vi "Init.vi"(8 "error in":errorcluster, 11 "Acquire Continuous Waveform Configuration in":refnum<class "Continuous Waveform Acq CFG.lvclass">) -> (0 "error out":errorcluster, 3 "Acquire Continuous Waveform Configuration out":refnum<class "Continuous Waveform Acq CFG.lvclass">)   [LabVIEW 2023, in "RIGOL DS1054.lvlib" / "Continuous Waveform Acq CFG.lvclass"]
uses:
  Continuous Waveform Acq CFG.lvclass
  <instrlib>/RIGOL DS1000 Series/RIGOL DS1000 Series.lvlib
  Configuration Base/Configuration Base.lvclass
  a845dea6-c2f2-4e03-ac8d-35208e94dd6c.vi
  <vilib>/ErrorRing/Error Ring.xnode
  <vilib>/Utility/error.llb/Error Cluster From Error Code.vi
  Scope VISA/Configuration/Scope VISA CFG.lvclass
  D:/git/HAL/Scope VISA/Configuration/Scope VISA CFG.lvclass
  D:/git/HAL/Scope Base/Configuration/Scope Base CFG.lvclass
  D:/git/HAL/Configuration Base/Configuration Base.lvclass
  D:/git/HAL/Interfaces/IConfigure/IConfigure.lvclass
  D:/git/HAL/Devices/Rigol DS1054/Configurations/Acquire Continuous Waveform/Continuous Waveform Acq CFG.lvclass
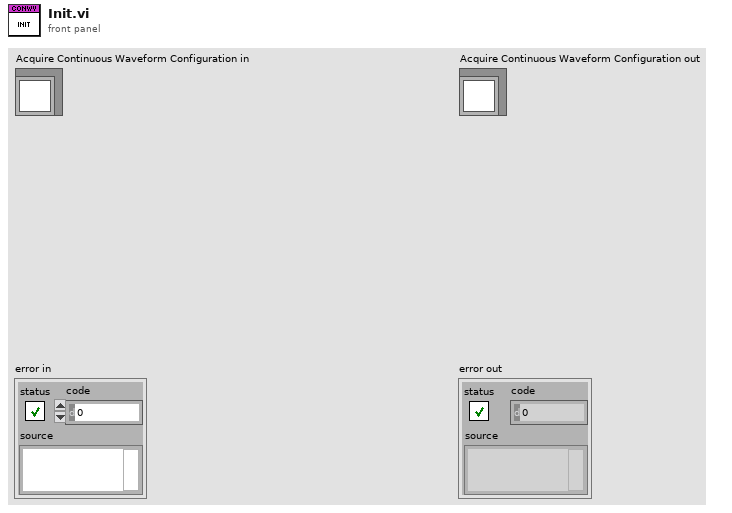
[diagram p1: front panel]
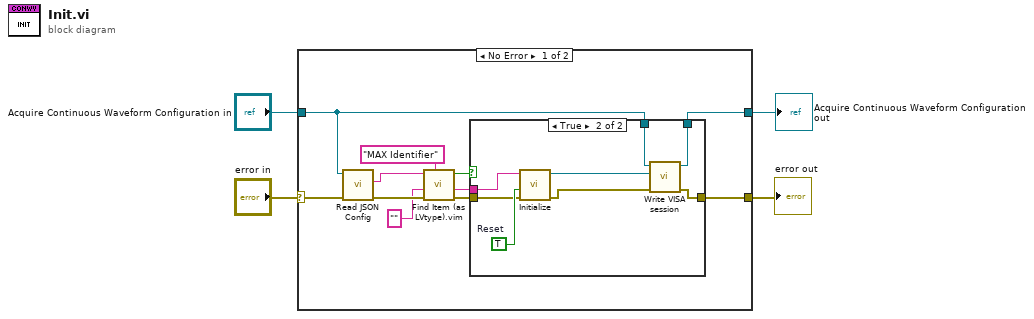
[diagram p0: block diagram]
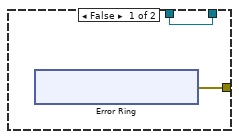
[diagram p2: hidden frame]
diagram:
  n1 = case shown="No Error" "error in" {
    selector: "error in" -> [w13 w32]
    tunnel: "Acquire Continuous Waveform Configuration in" -> [w5 w31]
    tunnel: [w15 w31] -> w3
    tunnel: [w14 w32] -> w1
    frame No Error {
      n2 = call "Read JSON Config.vi"("error in (no error)"=w13, "object in"=w5) -> ("error out"=w11:errorcluster, "<JSON>Config"=w12:string)  [unwired: 7 in, 1 out]
      n3 = call "Find Item (as LVtype).vim"("$Path or Item Name"="MAX Identifier", "error in (no error)"=w11, "Data Type and Default Value"="", "JSON"=w12) -> ("error out"=w6:errorcluster, "Data"=w8:string, "Found"=w7:bool)  [unwired: 4 in, 1 out]
      n4 = case shown="True" w7 {
        tunnel: [w16 w27] -> w15
        tunnel: [w17 w23] -> w14
        tunnel: w8 -> [_ w29]
        tunnel: w6 -> [_ w28]
        tunnel: w5 -> [w16 w26]
        frame False {
          n5 = xnode "Error Ring"() -> ("error out"=w17:errorcluster)
        }
        frame True {
          w30 = TRUE  # Reset
          n6 = call <instrlib>:"Initialize.vi"("error in (no error)"=w28, "Reset (True)"=w30, "VISA resource name"=w29) -> ("error out"=w24:errorcluster, "VISA resource name out"=w25:refnum<visa-resource-name>)  [unwired: 1 in, 6 out]
          n7 = call "Write VISA session.vi"("error in (no error)"=w24, "VISA session"=w25, "Scope VISA CFG in"=w26) -> ("error out"=w23:errorcluster, "Scope VISA CFG out"=w27:refnum<class "Continuous Waveform Acq CFG.lvclass">)  [unwired: 7 in]
        }
      }
    }
    frame Error {
    }
  }
  "error out" <- w1
  "Acquire Continuous Waveform Configuration out" <- w3
